vi "ROS_Master_lookupServiceReply.vi"(2 "Service":string, 3 "ROS_Master in":T1) -> (0 "XML":string)   [LabVIEW 2015]
doc: "Returns XML from registering a node with the master"
uses:
  ROS_Master.ctl
  ROS_Topic.ctl
  ROS_Node.ctl
  ROS_Service.ctl
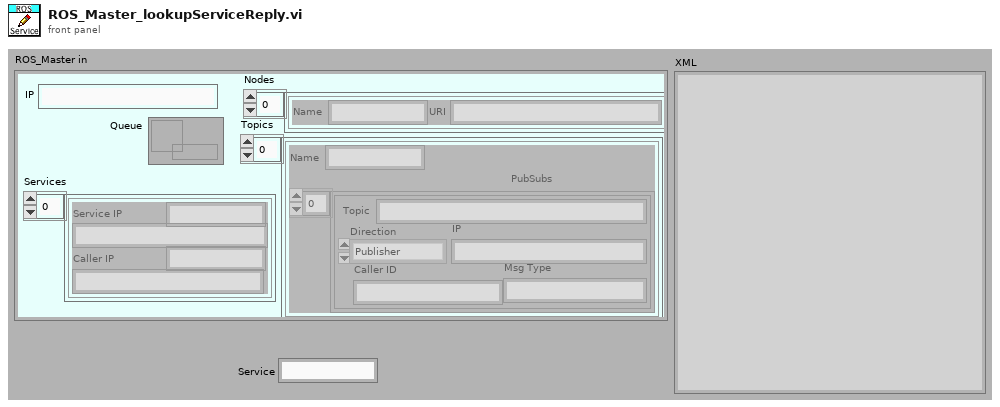
[diagram p1: front panel]
types:
  T1 = typedef "ROS_Master.ctl" = cluster{"IP":string, "Topics":cluster{"Name":string, "PubSubs":T2[]}[], "Nodes":T3[], "Services":T4[], "Queue":refnum<queue>}
  T2 = typedef "ROS_Topic.ctl" = cluster{"Caller ID":string, "IP":string, "Msg Type":string, "Direction":enum16{"Publisher", "Subscriber"}, "Topic":string}
  T3 = typedef "ROS_Node.ctl" = cluster{"Name":string, "URI":string}
  T4 = typedef "ROS_Service.ctl" = cluster{"Service":string, "Service IP":string, "Caller IP":string, "Caller ID":string}
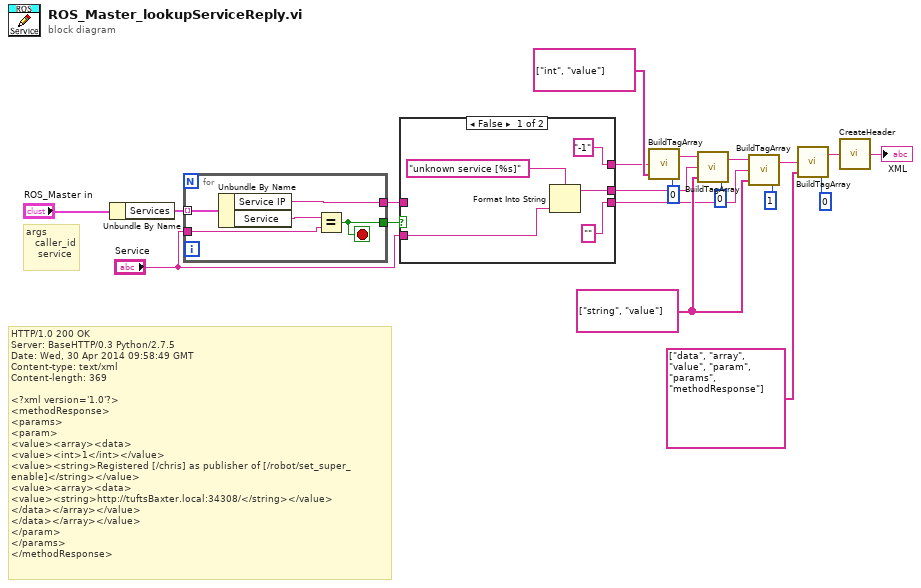
[diagram p0: block diagram]
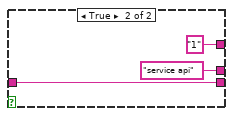
[diagram p2: hidden frame]
diagram:
  w11 = string[] ["string", "value"] ("tags")
  # "args\n   caller_id\n    service"
  # "HTTP/1.0 200 OK\nServer: BaseHTTP/0.3 Python/2.7.5\nDate: Wed, 30 Apr 2014 09:58:49 GMT\nContent-type: text/xml\nContent-length: 369\n\n<?xml version='1.0'?>\n<methodResponse>\n<params>\n<param>\n<value><array><data>\n<value><int>1</int></value>\n<value><string>Registered [/chris] as publisher of [/robot/set_super_enable]</string></value>\n<value><array><data>\n<value><string>http://tuftsBaxter.local:34308/</string></value>\n</data></array></value>\n</data></array></value>\n</param>\n</params>\n</methodResponse>"
  n1 = Unbundle By Name("ROS_Master in") -> ("Services"=w15:T4[])
  n2 = for {
    tunnel: w15 -> [w25] mode=indexing
    tunnel: "Service" -> [w23]
    tunnel: [w22] -> w14
    tunnel: [w21] -> w13
    stop <- w22 stop-if-true
    n3 = Unbundle By Name(w25) -> ("Service IP"=w21:string, "Service"=w24:string)
    n4 = Equal?(x=w24, y=w23) -> (x = y?=w22:bool)
  }
  n5 = case shown="False" w14 {
    tunnel: w13 -> [_ w32]
    tunnel: "Service" -> [w28 _]
    tunnel: ["-1" ("value") "1" ("value")] -> w9
    tunnel: ["" ("URI") w32] -> w8
    tunnel: [w27 "service api" ("value")] -> w7
    frame False {
      n6 = Format Into String(format string="unknown service [%s]", w28) -> (resulting string=w27:string)  [unwired: 2 in, 1 out]
    }
    frame True {
    }
  }
  n7 = call "BuildTagArray.vi"("Indent"=i8 0, "tags"=string[] ["int", "value"], "value"=w9) -> ("string out"=w19:string)  [unwired: 1 in]
  n8 = call "BuildTagArray.vi"("Indent"=i8 0, "tags"=w11, "value"=w7, "string in"=w19) -> ("string out"=w10:string)
  n9 = call "BuildTagArray.vi"("Indent"=i8 1, "tags"=w11, "value"=w8, "string in"=w10) -> ("string out"=w6:string)
  n10 = call "BuildTagArray.vi"("Indent"=i8 0, "tags"=string[] ["data", "array", "value", "param", "params", "methodResponse"], "value"=w6) -> ("string out"=w17:string)  [unwired: 1 in]
  n11 = call "CreateHeader.vi"("Content"=w17) -> ("XML"=→"XML":string)
